vi "U8 GUID to GUID.vi"(8 "error in (no error)":errorcluster, 11 "U8 GUID":u8[](array[numeric]) format="%.0x") -> (0 "error out":errorcluster, 3 "GUID In":string)   [LabVIEW 2021, in "DataTypes_CIF_U.lvlib"]
doc: "A GUID is a string representation of the hex values of 16 bytes. This converts a 16 element array of bytes to a GUID string with standard \"-\" separators."
uses:
  DataTypes_CIF_U.lvlib
  Typedef/Errors.ctl
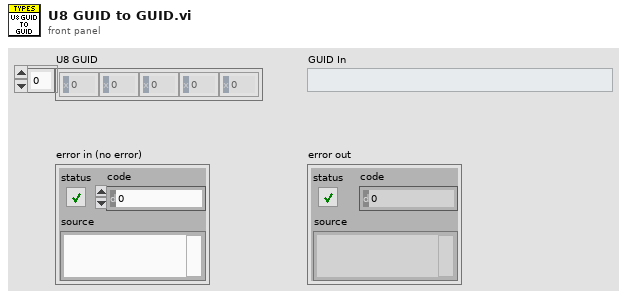
[diagram p1: front panel]
types:
  T1 = typedef "DataTypes_CIF_U.lvlib/Errors.ctl" = enum16{"Too few bytes", "Unsupported Type", "Invalid GUID"}
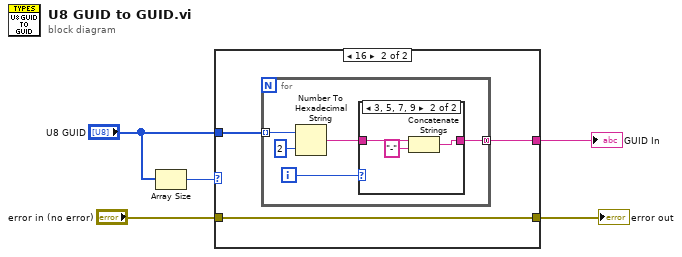
[diagram p0: block diagram]
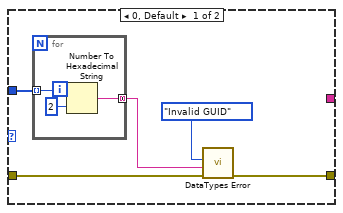
[diagram p2: hidden frame]
diagram:
  n1 = Array Size(array="U8 GUID") -> (size(s)=w3:i32)
  n2 = case shown="16" w3 {
    tunnel: "U8 GUID" -> [w8 w16]
    tunnel: [_ w15] -> w5
    tunnel: "error in (no error)" -> [w10 w14]
    tunnel: [w9 w14] -> w1
    frame 0, Default {
      n3 = for {
        tunnel: w8 -> [w13] mode=indexing
        tunnel: [w11] -> w6 mode=concatenating
        n4 = Number To Hexadecimal String(1:i16 2 ("width (-)"), 2:w13) -> (0:w11:string)
      }
      n5 = call "DataTypes Error.vi"("error in (no error)"=w10, "String to Append"=w6, "Error"=Errors."Invalid GUID") -> ("error out"=w9:errorcluster)  [unwired: 8 in]
    }
    frame 16 {
      n6 = for {
        tunnel: w16 -> [w21] mode=indexing
        tunnel: [w17] -> w15 mode=concatenating
        i -> [w18]
        n7 = Number To Hexadecimal String(1:i16 2 ("width (-)"), 2:w21) -> (0:w19:string)
        n8 = case shown="3, 5, 7, 9" w18 {
          tunnel: w19 -> [w22 w25]
          tunnel: [w22 w24] -> w17
          frame 0, Default {
          }
          frame 3, 5, 7, 9 {
            n9 = Concatenate Strings(w25, "-" ("string")) -> (w24:string)
          }
        }
      }
    }
  }
  "GUID In" <- w5
  "error out" <- w1
